vi "Read channels.vi"(8 "error in (no error)":errorcluster, 11 "Abstract Instrument in":refnum<class "Abstract Instrument.lvclass">) -> (0 "error out":errorcluster, 2 "channels":T1[](array[typedef]) {"Lower limit" format="%#_4p"; "Upper limit" format="%#_4p"}, 3 "Abstract Instrument out":refnum<class "Abstract Instrument.lvclass">)   [LabVIEW 2025, in "Abstract Engine.lvlib" / "Abstract Instrument.lvclass"]
uses:
  Abstract Instrument.lvclass
  Abstract Instrument.lvclass/Abstract Instrument.ctl
  Channel.ctl
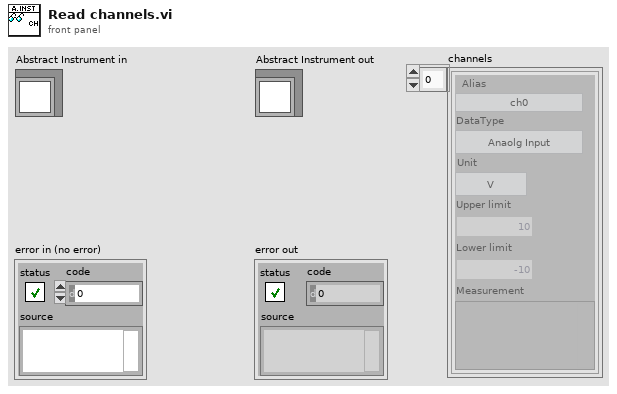
[diagram p1: front panel]
types:
  T1 = typedef "Abstract Engine.lvlib/Abstract Instrument.lvclass/Channel.ctl" = cluster{"Alias":string, "DataType":enum16{"Anaolg Input", "Waveform"}, "Unit":enum16{"---", "V", "A", "Ohm", "Hz", "uF", "degC", "deg"}, "Upper limit":dbl, "Lower limit":dbl, "Measurement":variant}
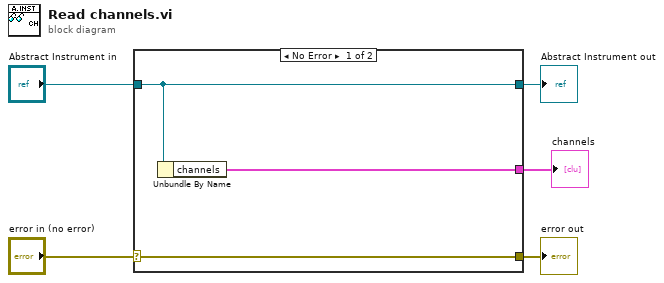
[diagram p0: block diagram]
diagram:
  n1 = case shown="No Error" "error in (no error)" {
    selector: "error in (no error)" -> [w8 w9]
    tunnel: [w8 w9] -> w4
    tunnel: [w7 w10] -> w2
    tunnel: "Abstract Instrument in" -> [w7 w10]
    tunnel: [w6 _] -> w1
    frame No Error {
      n2 = Unbundle By Name(w7) -> ("channels"=w6:T1[])
    }
    frame Error {
    }
  }
  "error out" <- w4
  "Abstract Instrument out" <- w2
  "channels" <- w1
